vi "database_connection_nowrite.vi"(5 "ODBC data source name":string="amrc_monitoring", 6 "error in (no error)":errorcluster, 7 "G1?":u32, 8 "current time":timestamp, 9 "data 2":dbl[](array[numeric]), 10 "Machine Data":T1={"Zload"="", "Yload"="", "Xload"="", "path_position"="", "Fovr"="", "SspeedOvr"="", "Program Name"="", "Program status"="", "Block of code being executed"="", "Line of code"="", "Machine availability"="", "Emergency status"="", "Controller mode"="", "Tool_id"="UNAVAILABLE"}, 11 "Machine type":string) -> (3 "error out":errorcluster)   [LabVIEW 2017]
uses:
  <vilib>/addons/database/Connection.llb/DB Tools Open Connec (String).vi
  <vilib>/addons/database/NI_Database_API.lvlib
panel:
  out "resulting string":string
  out "size(s)":i32
  out "concatenated string 5":string
  out "concatenated string 4":string
  out "concatenated string 3":string
  out "concatenated string 2":string
  out "concatenated string":string
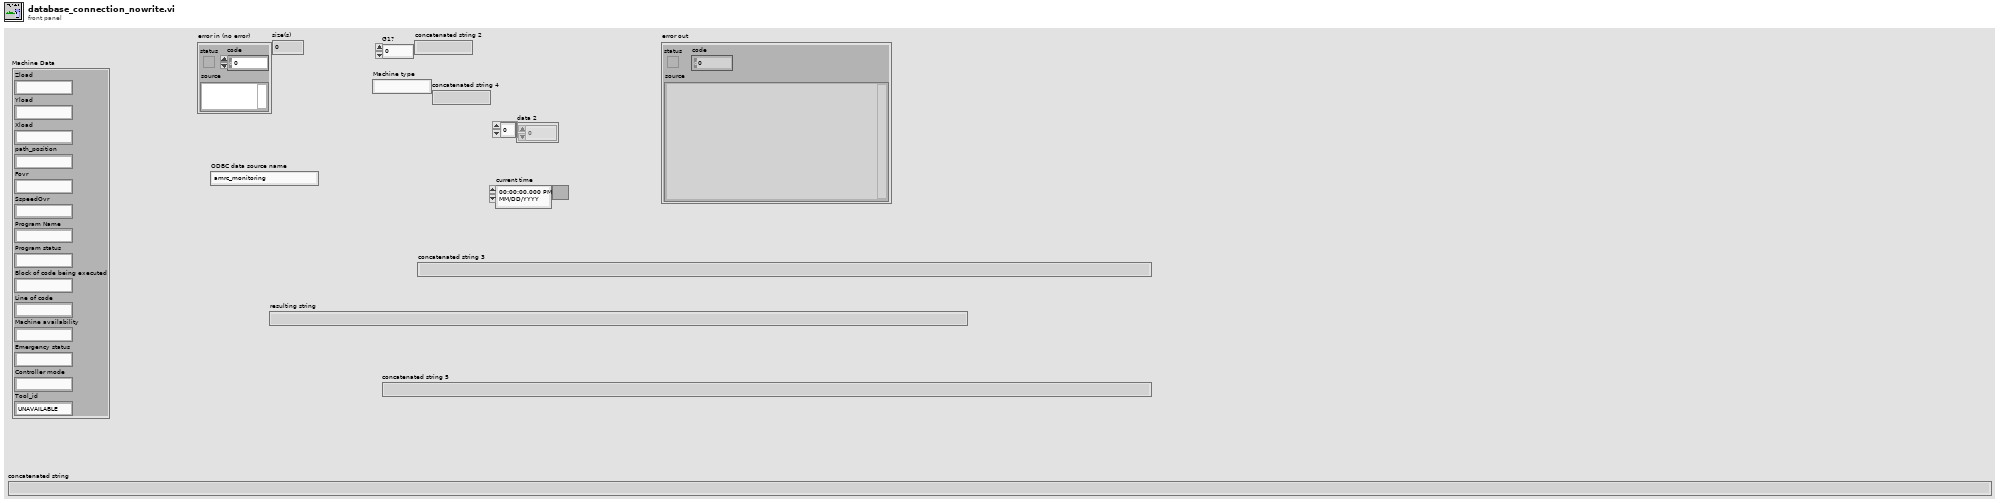
[diagram p1: front panel]
types:
  T1 = cluster{"Zload":string, "Yload":string, "Xload":string, "path_position":string, "Fovr":string, "SspeedOvr":string, "Program Name":string, "Program status":string, "Block of code being executed":string, "Line of code":string, "Machine availability":string, "Emergency status":string, "Controller mode":string, "Tool_id":string}
  T2 = typedef "NI_Database_API.lvlib/Conn ObjectReference.ctl" = refnum<k1>
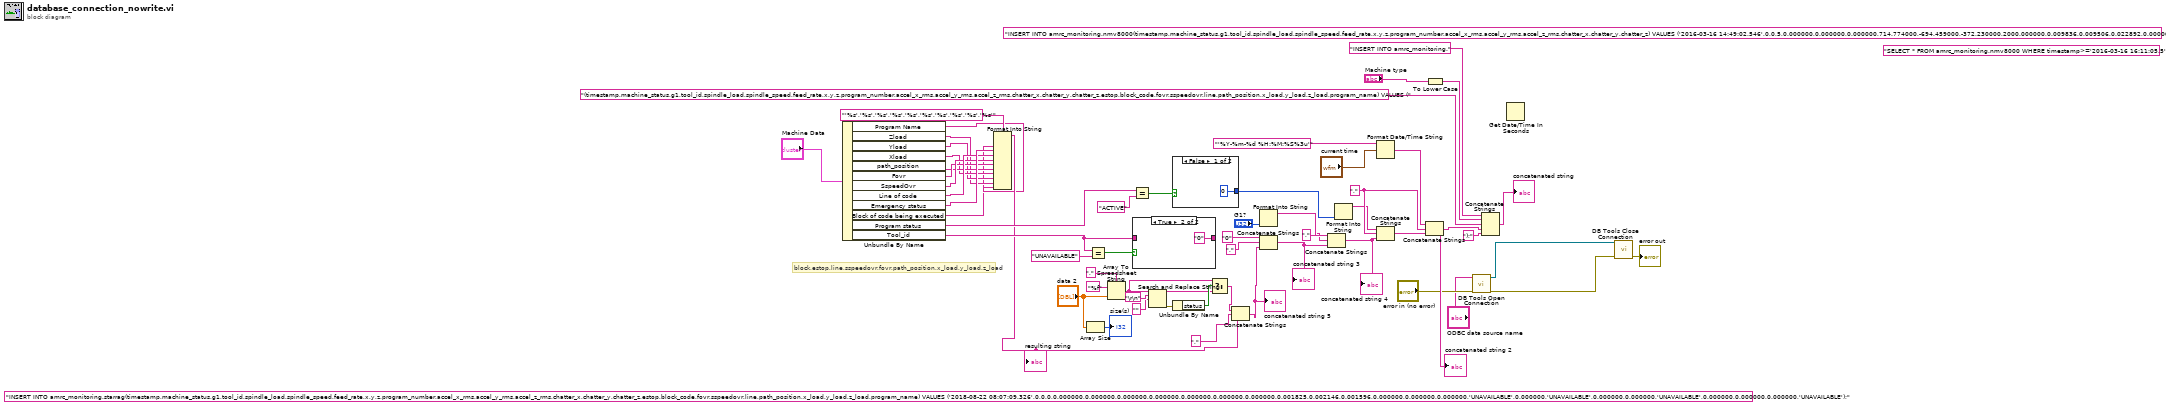
[diagram p0: block diagram]
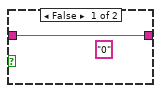
[diagram p2: hidden frame]
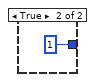
[diagram p3: hidden frame]
diagram:
  (unwired) "INSERT INTO amrc_monitoring.starrag(timestamp,machine_status,g1,tool_id,spindle_load,spindle_speed,feed_rate,x,y,z,program_number,accel_x_rms,accel_y_rms,accel_z_rms,chatter_x,chatter_y,chatter_z,estop,block_code,fovr,sspeedovr,line,path_position,x_load,y_load,z_load,program_name) VALUES ('2018-08-22 08:07:09.326',0,0,0,0.000000,0.000000,0.000000,0.000000,0.000000,0.000000,0.000000,0.001825,0.002146,0.001596,0.000000,0.000000,0.000000,'UNAVAILABLE',0.000000,'UNAVAILABLE',0.000000,0.000000,'UNAVAILABLE',0.000000,0.000000,0.000000,'UNAVAILABLE');" ("string")
  w43 = "," ("string")
  (unwired) "SELECT * FROM amrc_monitoring.nmv8000 WHERE timestamp>='2016-03-16 16:11:05.5' " ("SQL query")
  (unwired) "INSERT INTO amrc_monitoring.nmv8000(timestamp,machine_status,g1,tool_id,spindle_load,spindle_speed,feed_rate,x,y,z,program_number,accel_x_rms,accel_y_rms,accel_z_rms,chatter_x,chatter_y,chatter_z) VALUES ('2016-03-16 14:49:02.546',0,0,5,0.000000,0.000000,0.000000,714.774000,-694.459000,-372.230000,2000.000000,0.009836,0.009506,0.022892,0.000000,1.000000,0.000000);" ("SQL query")
  # "block,estop,line,sspeedovr,fovr,path_position,x_load,y_load,z_load"
  n1 = Unbundle By Name("Machine Data") -> ("Program Name"=w13:string, "Zload"=w19:string, "Yload"=w20:string, "Xload"=w21:string, "path_position"=w22:string, "Fovr"=w23:string, "SspeedOvr"=w24:string, "Line of code"=w25:string, "Emergency status"=w26:string, "Block of code being executed"=w9:string, "Program status"=w55:string, "Tool_id"=w50:string)
  n2 = Format Into String(format string="'%s','%s','%s','%s','%s','%s','%s','%s','%s','%s'", w9, w26, w25, w24, w23, w22, w21, w20, w19, w13) -> (resulting string=w16:string)  [unwired: 2 in, 1 out]
  "resulting string" <- w16
  n3 = Array Size(array="data 2") -> (size(s)=→"size(s)":i32)
  n4 = Equal?(x=w50, y="UNAVAILABLE") -> (x = y?=w51:bool)
  n5 = Array To Spreadsheet String(delimiter (Tab)=",", array="data 2", 3:"%f" ("format string")) -> (spreadsheet string=w34:string)
  n6 = case shown="True" w51 {
    tunnel: w50 -> [w59 _]
    tunnel: [w59 "0"] -> _
    frame False {
      (unwired) "0"
    }
    frame True {
    }
  }
  n7 = Equal?(x=w55, y="ACTIVE") -> (x = y?=w53:bool)
  n8 = Search and Replace String(input string=w34, search string="\r\n", replace string="" ("replace string (\"\")")) -> (result string=w35:string, error out=w37:errorcluster)  [unwired: 5 in, 2 out]
  n9 = case shown="False" w53 {
    tunnel: [0 1] -> w52
    frame False {
    }
    frame True {
    }
  }
  n10 = Unbundle By Name(w37) -> ("status"=w36:bool)
  n11 = Select(t=w34, s=w36, f=w35) -> (s? t:f=w15:string)
  n12 = Concatenate Strings(w15, "," ("string"), w16) -> (w14:string)
  "concatenated string 5" <- w14
  n13 = Format Into String("G1?") -> (resulting string=w47:string)  [unwired: 3 in, 1 out]
  n14 = Concatenate Strings("0", "," ("string"), w14) -> (w7:string)
  "concatenated string 3" <- w7
  n15 = Concatenate Strings(w47, "," ("string"), w7) -> (w12:string)
  "concatenated string 4" <- w12
  n16 = Format Into String(w52) -> (resulting string=w41:string)  [unwired: 3 in, 1 out]
  n17 = Concatenate Strings(w41, w43, w12) -> (w44:string)
  n18 = Format Date/Time String(time format string (%c)="'%Y-%m-%d %H:%M:%S%3u'", seconds (now)="current time") -> (date/time string=w42:string)  [unwired: 1 in]
  n19 = Concatenate Strings(w42, w43, w44) -> (w40:string)
  "concatenated string 2" <- w40
  n20 = To Lower Case(string="Machine type") -> (all lower case string=w31:string)
  n21 = call-poly <vilib>:"DB Tools Open Connection.vi"("error in (no error)"="error in (no error)", "connection information"="ODBC data source name") -> ("error out"=w2:errorcluster, "connection reference"=w1:T2)  [unwired: 6 in]
  n22 = Concatenate Strings("INSERT INTO amrc_monitoring." ("string"), w31, "(timestamp,machine_status,g1,tool_id,spindle_load,spindle_speed,feed_rate,x,y,z,program_number,accel_x_rms,accel_y_rms,accel_z_rms,chatter_x,chatter_y,chatter_z,estop,block_code,fovr,sspeedovr,line,path_position,x_load,y_load,z_load,program_name) VALUES (" ("string"), w40, ");" ("string")) -> (→"concatenated string":string)
  n23 = Get Date/Time In Seconds() -> ()  [unwired: 1 out]
  n24 = call <vilib>:"DB Tools Close Connection.vi"("error in (no error)"=w2, "connection reference"=w1) -> ("error out"=→"error out":errorcluster)  [unwired: 5 in]
